vi "MIMIC Commands.vi"(0 "VISA resource name":refnum<visa-resource-name>="COM1", 1 "Baud Rate":dbl, 4 "Verify CheckSum":bool=TRUE, 5 "Read COM Port":bool=TRUE, 6 "Write to COM Port":bool=TRUE, 7 "Add CheckSum":bool=TRUE, 12 "String To Write":string="*IDN?", 13 "Send Command":bool, 14 "ACK HEX String":string="*IDN?", 15 "ACK":bool, 17 "Response: bytes to\n read":u32=5, 18 "Response":bool, 19 "ACK: bytes to read":u32=5) -> (2 "Response RECEIVE ERROR":bool, 3 "ACK RECEIVE Error":bool, 8 "Command SENT Error":bool, 9 "Open Comport Error":bool, 10 "CheckSum SUCCESS":bool, 11 "Response HEX String":string, 16 "Close Comport Error":bool)   [LabVIEW 2014]
doc: "The Basic Serial Read and Write example performs a Serial Port Read, a Serial Port Write, or a combination of these actions. The user selects the actions (read or write) on the front panel. If both are selected, the VI will write the data first, read data, and then close the VISA session that is opened to the port. This VI will wait until the specified number of bytes is received at the port. Only the number of bytes specified will be read.\n\nINSTRUCTIONS:\n1) Select the serial resource and configuration parameters (baud rate, data bits, parity, stop bits, flow control).\n2) Select the operations to be performed. \n3) Connect the serial port to your device. If no device is available, perform a loopback test by doing one of the following. Short pins 2 and 3 on a RS-232 cable or short pin 4 to pin 8 and pin 5 to pin 9 on a RS-485/422 cable. \n4) Run the VI to see the data read. (The \"read string\" will match the \"string to write\" if a loopback test was performed.)\n\nNote: The parameters set for the serial port must match the parameters of the connected instrument or device. In this example, the bytes to read parameter specifies the number of bytes that the serial port reads. If there were more bytes at the port than the number specified in bytes to read, those bytes would not be read. Also, if you specify to read more bytes than the number of bytes actually read, you might receive a timeout error message.\n\nOn the block diagram, the Configure Serial Port VI sets the configuration parameters. The front panel displays the controls used to configure the basic parameters, such as baud rate, data bits, and parity. Constants configure the other parameters the user probably does not need set. After the VISA Configure Serial Port VI opens the VISA session and configures the port, the VI passes the VISA resource name to other VIs that perform operations on that VISA resource. The VISA Write function sends a command to the serial device and the VISA Read function returns data based on the command. The VISA Close function then closes the reference to the serial device. It is important to close the reference; otherwise communication through with that port through protocols other than VISA might not be possible."
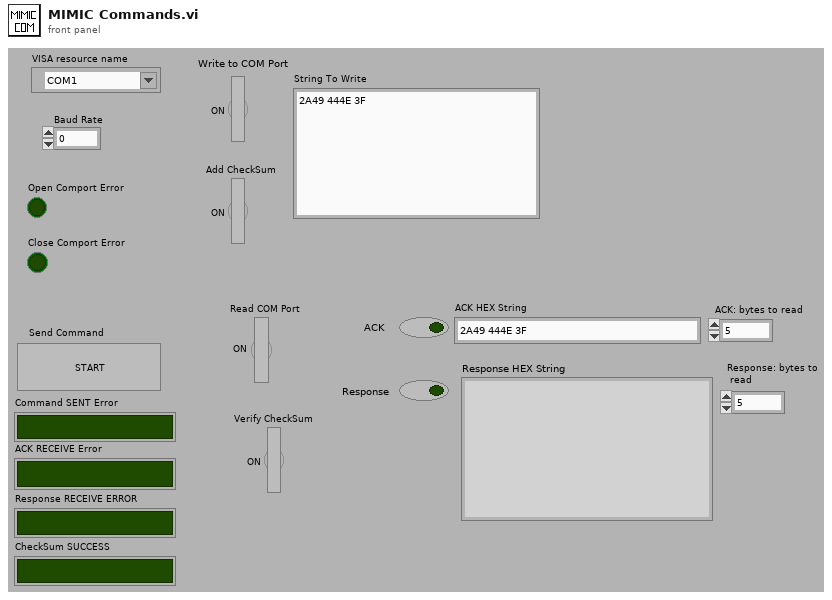
[diagram p1: front panel]
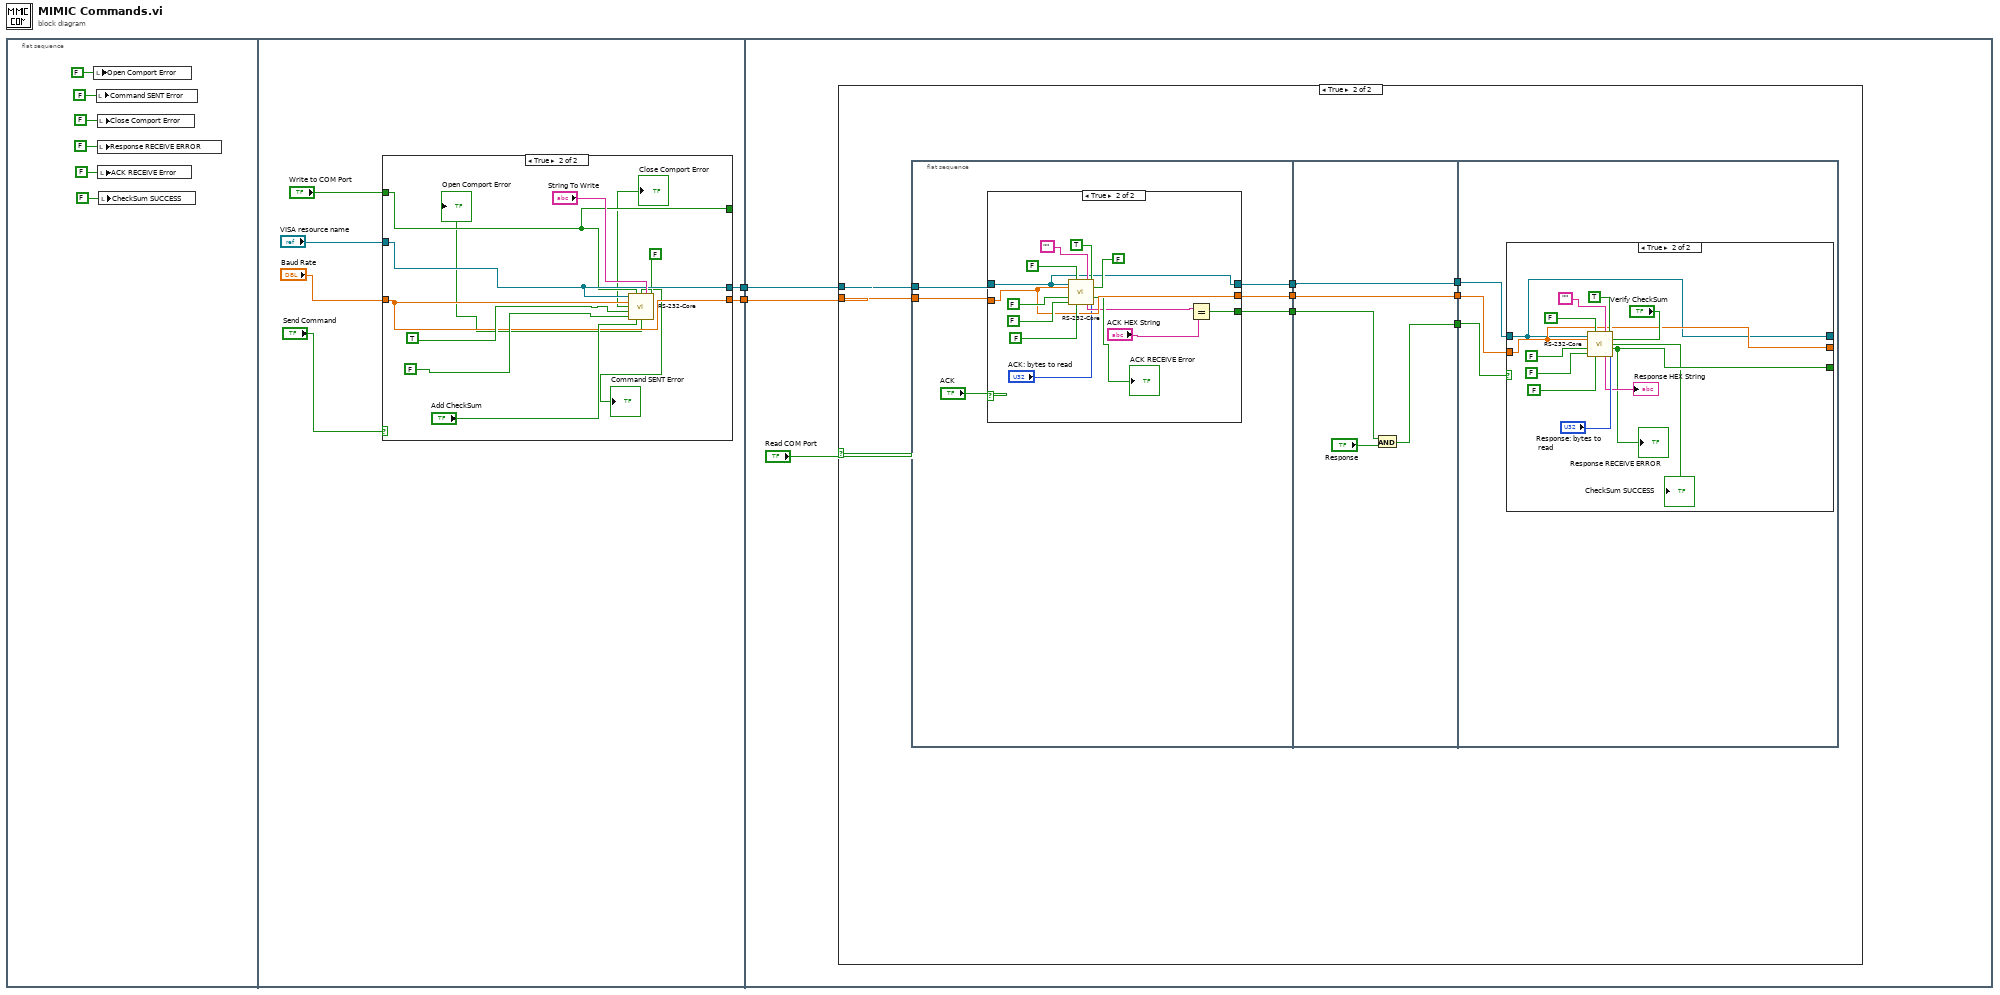
[diagram p0: block diagram]
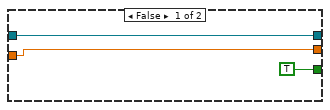
[diagram p4: hidden frame]
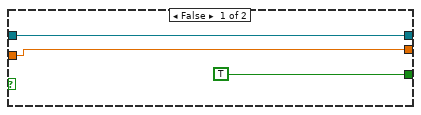
[diagram p5: hidden frame]
diagram:
  n1 = flat-sequence {
    tunnel: [w11] -> w2
    tunnel: [w10] -> w1
    tunnel: w2 -> [w30]
    tunnel: w1 -> [w29]
    frame #0 {
      n2 = local write "Open Comport Error"(FALSE ("Open Comport Error")) -> ()
      n3 = local write "Command SENT Error"(FALSE ("Command SENT Error")) -> ()
      n4 = local write "Close Comport Error"(FALSE ("Close Comport Error")) -> ()
      n5 = local write "Response RECEIVE ERROR"(FALSE ("Response RECEIVE ERROR")) -> ()
      n6 = local write "ACK RECEIVE Error"(FALSE ("ACK RECEIVE Error")) -> ()
      n7 = local write "CheckSum SUCCESS"(FALSE ("CheckSum SUCCESS")) -> ()
    }
    frame #1 {
      n8 = case shown="True" "Send Command" {
        tunnel: "VISA resource name" -> [w17 w24]
        tunnel: "Baud Rate" -> [w16 w23]
        tunnel: "Write to COM Port" -> [w15 w22]
        tunnel: [w17 w24] -> w11
        tunnel: [w16 w23] -> w10
        tunnel: [w15 w22] -> _
        frame False {
        }
        frame True {
          n9 = call "RS-232-Core.vi"("VISA resource name"=w24, "Write to COM Port"=w22, "String To Write"="String To Write", "Read COM Port"=FALSE, "baud rate"=w23, "Initialize COMPort"=TRUE, "Close COMPort"=FALSE, "Add CheckSum"="Add CheckSum") -> ("Sent?"=→"Command SENT Error":bool, "Close"=→"Close Comport Error":bool, "Open?"=→"Open Comport Error":bool)  [unwired: 2 in, 3 out]
        }
      }
    }
    frame #2 {
      n10 = case shown="True" "Read COM Port" {
        tunnel: w30 -> [_ w39]
        tunnel: w29 -> [_ w38]
        frame False {
        }
        frame True {
          n11 = flat-sequence {
            tunnel: w39 -> [w44]
            tunnel: w38 -> [w43]
            tunnel: [w42] -> w37
            tunnel: [w41] -> w36
            tunnel: [w40] -> w35
            tunnel: w37 -> [w65]
            tunnel: w36 -> [w64]
            tunnel: w35 -> [w66]
            tunnel: [w65] -> w34
            tunnel: [w64] -> w33
            tunnel: [w63] -> w32
            tunnel: w34 -> [w68]
            tunnel: w33 -> [w69]
            tunnel: w32 -> [w70]
            frame #0 {
              n12 = case shown="True" "ACK" {
                tunnel: w44 -> [w48 w53]
                tunnel: w43 -> [w47 w52]
                tunnel: [TRUE w54] -> w40
                tunnel: [w48 w53] -> w42
                tunnel: [w47 w52] -> w41
                frame False {
                }
                frame True {
                  n13 = call "RS-232-Core.vi"("VISA resource name"=w53, "Write to COM Port"=FALSE, "String To Write"="", "Read COM Port"=TRUE, "baud rate"=w52, "Verify CheckSum"=FALSE, "Initialize COMPort"=FALSE, "Close COMPort"=FALSE, "Add CheckSum"=FALSE, "bytes to read"="ACK: bytes to read") -> ("Response?"=→"ACK RECEIVE Error":bool, "Read String"=w50:string)  [unwired: 4 out]
                  n14 = Equal?(x=w50, y="ACK HEX String") -> (x = y?=w54:bool)
                }
              }
            }
            frame #1 {
              n15 = And(x=w66, y="Response") -> (x .and. y?=w63:bool)
            }
            frame #2 {
              n16 = case shown="True" w70 {
                tunnel: w68 -> [w73 w76]
                tunnel: w69 -> [w72 w77]
                tunnel: [TRUE w75] -> _
                tunnel: [w73 w76] -> _
                tunnel: [w72 w77] -> _
                frame False {
                }
                frame True {
                  n17 = call "RS-232-Core.vi"("VISA resource name"=w76, "Write to COM Port"=FALSE, "String To Write"="", "Read COM Port"=TRUE, "baud rate"=w77, "Verify CheckSum"="Verify CheckSum", "Initialize COMPort"=FALSE, "Close COMPort"=FALSE, "Add CheckSum"=FALSE, "bytes to read"="Response: bytes to\n read") -> ("CheckSum?"=→"CheckSum SUCCESS":bool, "Response?"=w75:bool, "Read String"=→"Response HEX String":string)  [unwired: 3 out]
                  "Response RECEIVE ERROR" <- w75
                }
              }
            }
          }
        }
      }
    }
  }
